vi "Get velocity.vi"(0 "Zaber":T1={"Serial port handle"="", "Axis"="", "Controller #"=0, "Min position"=0.0, "Max position"=0.0, "Min velocity"=0.0, "Max velocity"=0.0, "Firmware"="", "Device ID"=0, "Variable event"=refnum, "Variable ref"=refnum, "Resolution, usteps/step"=0, "Serial port semaphore"=refnum, "Joystick buttons"={"MinDir"=1, "MaxDir"=2, "MedSpeed"=5, "HighSpeed"=6}} {"Joystick buttons"."HighSpeed" min=1 max=25 step=1; "Joystick buttons"."MedSpeed" min=1 max=25 step=1; "Joystick buttons"."MaxDir" min=1 max=25 step=1; "Joystick buttons"."MinDir" min=1 max=25 step=1}, 5 "error in":errorcluster) -> (14 "Zaber out":T1={"Serial port handle"="", "Axis"="", "Controller #"=0, "Min position"=0.0, "Max position"=0.0, "Min velocity"=0.0, "Max velocity"=0.0, "Firmware"="", "Device ID"=0, "Variable event"=refnum, "Variable ref"=refnum, "Resolution, usteps/step"=0, "Serial port semaphore"=refnum, "Joystick buttons"={"MinDir"=1, "MaxDir"=2, "MedSpeed"=5, "HighSpeed"=6}} {"Joystick buttons"."HighSpeed" min=1 max=25 step=1; "Joystick buttons"."MedSpeed" min=1 max=25 step=1; "Joystick buttons"."MaxDir" min=1 max=25 step=1; "Joystick buttons"."MinDir" min=1 max=25 step=1}, 16 "Velocity, mm/s":dbl, 17 "Velocity, counts":i32, 19 "error out":errorcluster)   [LabVIEW 2018]
uses:
  Zaber.ctl
  GenericDataEvent/GenericEvent.ctl
  ZaberVariables.ctl
  CommandZaber.ctl
  GenericDataEvent/GenericData.ctl
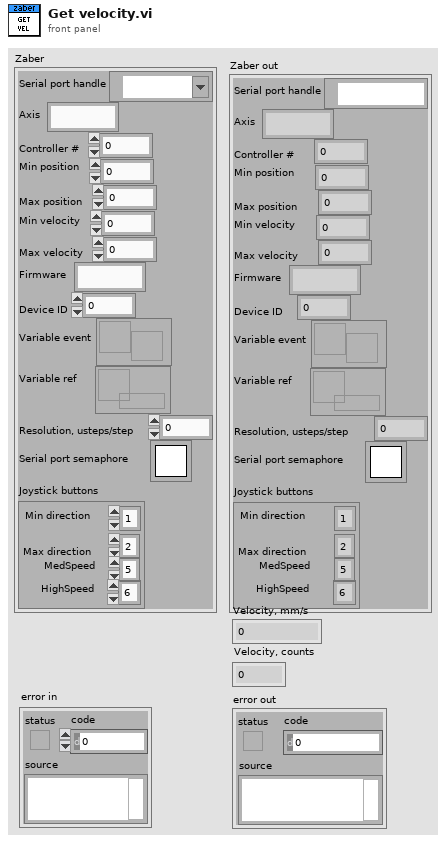
[diagram p1: front panel]
types:
  T1 = typedef "Zaber.ctl" = cluster{"Serial port handle":refnum<visa-resource-name>, "Axis":string, "Controller #":u8, "Min position":dbl, "Max position":dbl, "Min velocity":dbl, "Max velocity":dbl, "Firmware":string, "Device ID":i32, "Variable event":T2, "Variable ref":refnum<data-value>, "Resolution, usteps/step":i32, "Serial port semaphore":T3, "Joystick buttons":cluster{"MinDir":i32, "MaxDir":i32, "MedSpeed":i32, "HighSpeed":i32}}
  T2 = typedef "GenericEvent.ctl" = refnum<user-event>
  T3 = typedef "Semaphore RefNum" = refnum<k1>
  T4 = typedef "CommandZaber.ctl" = cluster{"Command":u8, "Data":i32}
  T5 = typedef "ZaberVariables.ctl" = cluster{"Position":i32, "Speed":i32, "Min soft position":dbl, "Max soft position":dbl, "Accelaration":i32}
  T6 = typedef "GenericData.ctl" = cluster{"Name":string, "Data":variant}
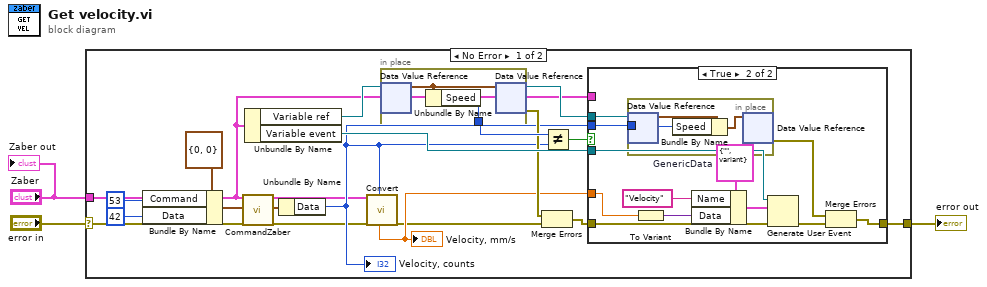
[diagram p0: block diagram]
diagram:
  n1 = case shown="No Error" "error in" {
    selector: "error in" -> [w19 w42]
    tunnel: [w17 w42] -> w2
    tunnel: "Zaber" -> [w9 _]
    frame No Error {
      n2 = Bundle By Name(cluster=T4 {"Command"=0, "Data"=0} ("Command"), "Command"=53 ("Data"), "Data"=42) -> (w22:T4)
      n3 = call "CommandZaber.vi"("Zaber"=w9, "Command"=w22, "error in"=w19) -> ("Zaber out"=w4:T1, "Answer"=w18:T4, "error out"=w6:errorcluster)  [unwired: 13 in, 1 out]
      n4 = Unbundle By Name(w9) -> ("Variable ref"=w15:refnum<data-value>, "Variable event"=w16:T2)
      n5 = Unbundle By Name(w18) -> ("Data"=w8:i32)
      "Velocity, counts" <- w8
      n6 = call "Convert.vi"("Zaber"=w4, "error in"=w6, "Velocity, counts"=w8) -> ("Velocity, mm/s"=w7:dbl, "error out"=w5:errorcluster)  [unwired: 8 in, 7 out]
      "Velocity, mm/s" <- w7
      n7 = in-place {
        in-place-border: [w24] -> w12
        n8 = in-place-dvr #1(w15) -> (w25:T5)  [unwired: 1 out]
        n9 = Unbundle By Name(w25) -> ("Speed"=w24:i32)
        n10 = in-place-dvr #1(w25) -> (w14:refnum<data-value>, w10:errorcluster)
      }
      n11 = Merge Errors(w10, w5) -> (w11:errorcluster)
      n12 = Not Equal?(x=w12, y=w8) -> (x != y?=w13:bool)
      n13 = case shown="True" w13 {
        tunnel: w11 -> [w26 w38]
        tunnel: [w26 w27] -> w17
        tunnel: w7 -> [_ w33]
        tunnel: w16 -> [_ w37]
        tunnel: w9 -> [_ _]
        tunnel: w8 -> [_ w30]
        tunnel: w14 -> [_ w31]
        frame False {
        }
        frame True {
          w36 = T6 {"Name"="", "Data"=variant}  # GenericData
          n14 = in-place {
            in-place-border: w30 -> [w40]
            n15 = in-place-dvr #2(w31) -> (w41:T5)  [unwired: 1 out]
            n16 = Bundle By Name(cluster=w41, "Speed"=w40) -> (w39:T5)
            n17 = in-place-dvr #2(w39) -> (w29:errorcluster)  [unwired: 1 out]
          }
          n18 = To Variant(anything=w33) -> (Variant=w32:variant)
          n19 = Bundle By Name(cluster=w36, "Name"="Velocity", "Data"=w32) -> (w34:T6)
          n20 = Generate User Event(user event=w37, event data cluster=w34, error in=w38) -> (error out=w28:errorcluster)  [unwired: 1 in, 1 out]
          n21 = Merge Errors(w29, w28) -> (w27:errorcluster)
        }
      }
    }
    frame Error {
    }
  }
  "error out" <- w2
  "Zaber out" <- "Zaber"
